vi "Fc_start_record.vi"(0 "Trace names":refnum<vi>, 1 "Start record?":refnum<vi>, 2 "Samples X Signal":u32, 3 "Global Mode":enum32{"Item 0", "Item 1"}(ring), 5 "Refresh \ntime (ms)":i32, 7 "total samples?":refnum<vi>, 9 "status+start record":bool, 11 "error in (no error)":errorcluster, 14 "Class TCP in":T1) -> (4 "Class TCP out":T1, 15 "error out":errorcluster)   [LabVIEW 2021]
doc: "This function starts the record of the signals in the application."
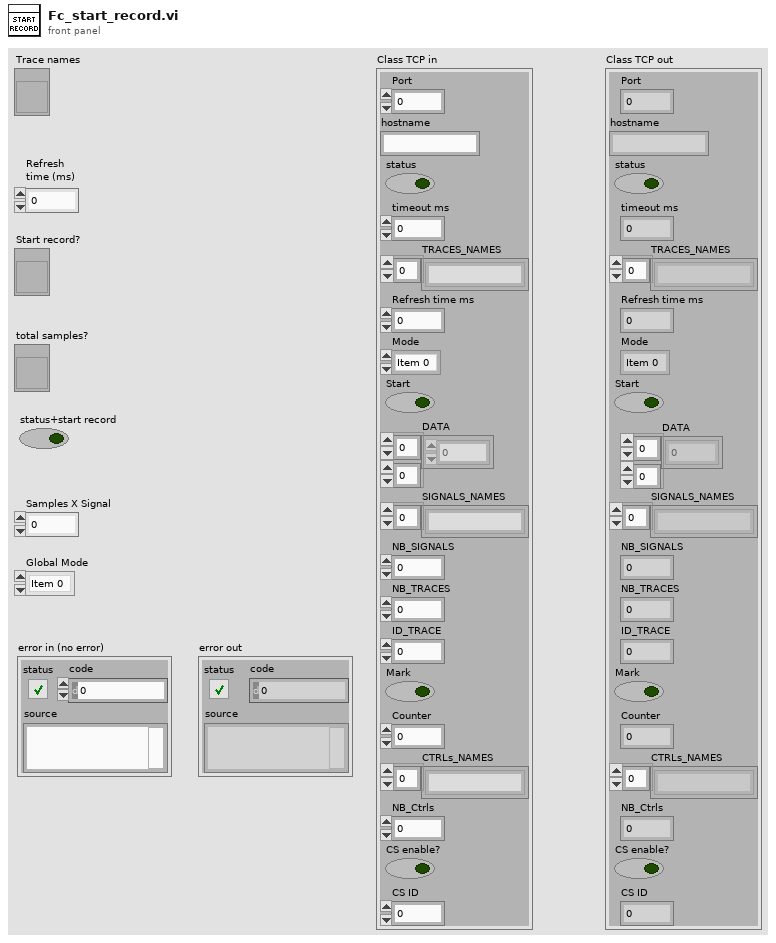
[diagram p1: front panel]
types:
  T1 = cluster{"Port":i32, "hostname":string, "status":bool, "timeout ms":i32, "TRACES_NAMES":string[], "Refresh time ms":i32, "Mode":enum32{"Item 0", "Item 1"}, "Start":bool, "DATA":sgl[][], "SIGNALS_NAMES":string[], "NB_SIGNALS":i32, "NB_TRACES":i32, "ID_TRACE":i32, "Mark":bool, "Counter":i32, "CTRLs_NAMES":string[], "NB_Ctrls":i32, "CS enable?":bool, "CS ID":i32}
  T2 = cluster{"TRACE_SIZE":i32, "CS_ID":i32, "TRACE ID":i32, "CMD":i32, "DATA(M)":i32}
  T3 = cluster{"timeout ms":i32, "remote port":u16, "Address":string}
  T4 = cluster{"SIZE":i32, " TRACE DATA":sgl[], "TRACE_SIZE":i32, "NB_TRACES":i32, "NB_TRACED_SIGNALS":i32, "NAMES TRACED SIGNALS":string[], "NAMES TRACES":string[], "CS STATUS":i32, "NB_CSs":i32, "NAMES CSs":string[], "DATA (M)":sgl[], "CMD":i32}
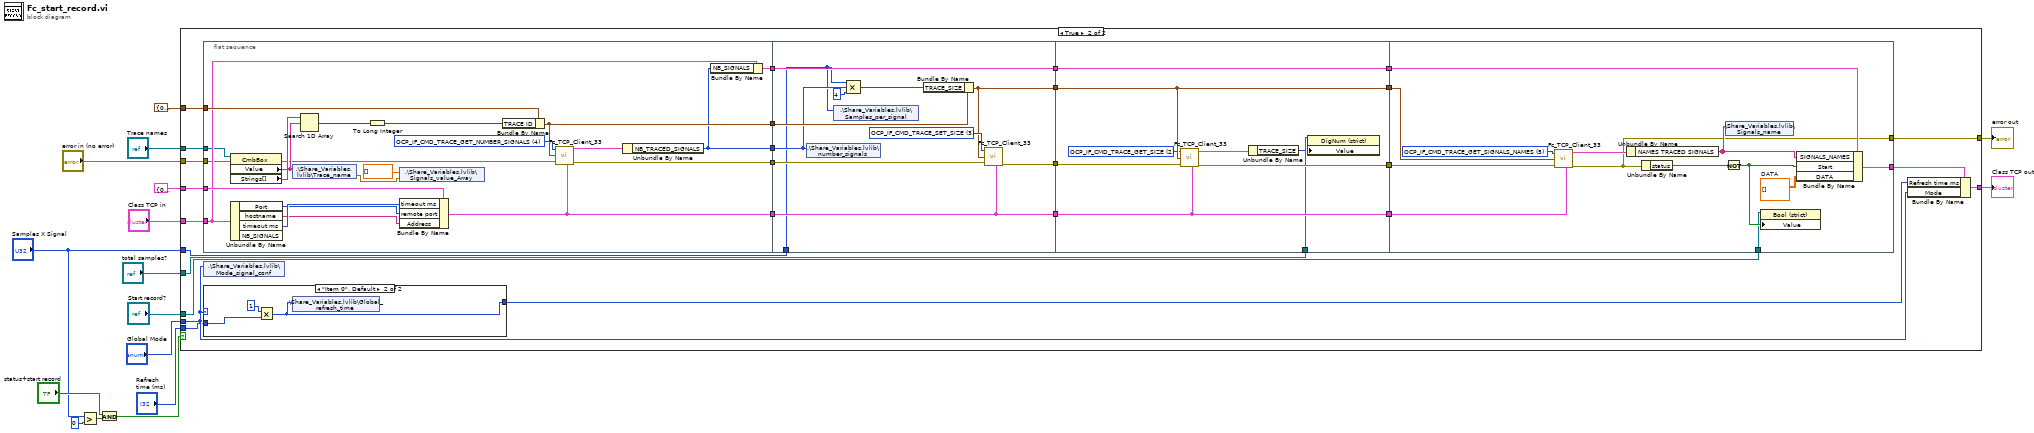
[diagram p0: block diagram]
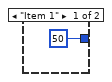
[diagram p3: hidden frame]
diagram:
  n1 = Greater?(x="Samples X Signal", y=0) -> (0:w2:bool)
  n2 = And(x="status+start record", y=w2) -> (x .and. y?=w1:bool)
  n3 = case shown="True" w1 {
    tunnel: "Class TCP in" -> [w18 w43]
    tunnel: [w18 w45] -> w12
    tunnel: T3 {"timeout ms"=0, "remote port"=0, "Address"=""} ("Comunication Cluster") -> [_ w41]
    tunnel: T2 {"TRACE_SIZE"=0, "CS_ID"=0, "TRACE ID"=0, "CMD"=0, "DATA(M)"=0} ("Input Cluster") -> [_ w40]
    tunnel: "Samples X Signal" -> [_ w39]
    tunnel: "Global Mode" -> [_ w38]
    tunnel: "Refresh \ntime (ms)" -> [_ w37]
    tunnel: "Trace names" -> [_ w36]
    tunnel: "Start record?" -> [_ w35]
    tunnel: "total samples?" -> [_ w34]
    tunnel: [w17 w33] -> w7
    tunnel: "error in (no error)" -> [w17 w32]
    frame False {
    }
    frame True {
      n4 = flat-sequence {
        tunnel: w43 -> [w51]
        tunnel: [w64] -> w31
        tunnel: [w50] -> w30
        tunnel: [w58] -> w29
        tunnel: [w53] -> w28
        tunnel: w41 -> [w57]
        tunnel: w40 -> [w56]
        tunnel: [w49] -> w27
        tunnel: w36 -> [w47]
        tunnel: w32 -> [w46]
        tunnel: w31 -> [w77]
        tunnel: [w76] -> w26
        tunnel: w30 -> [w78]
        tunnel: [w78] -> w25
        tunnel: w29 -> [w73]
        tunnel: w28 -> [w74]
        tunnel: [w74] -> w24
        tunnel: w27 -> [w72]
        tunnel: w39 -> [w68]
        tunnel: [w69] -> w23
        tunnel: w26 -> [w86]
        tunnel: [w85] -> w21
        tunnel: w25 -> [w87]
        tunnel: [w87] -> w22
        tunnel: [w84] -> w19
        tunnel: w24 -> [w83]
        tunnel: [w83] -> w20
        tunnel: w23 -> [w84]
        tunnel: w34 -> [w82]
        tunnel: w22 -> [w100]
        tunnel: [w99] -> w42
        tunnel: w21 -> [w97]
        tunnel: w20 -> [w95]
        tunnel: w19 -> [w94]
        tunnel: w35 -> [w89]
        tunnel: [w88] -> w33
        frame #0 {
          w63 = 4 items=["OCP_IF_CMD_TRACE_READ", "OCP_IF_CMD_TRACE_RESET", "OCP_IF_CMD_TRACE_GET_SIZE", "OCP_IF_CMD_TRACE_SET_SIZE", "OCP_IF_CMD_TRACE_GET_NUMBER_SIGNALS", "OCP_IF_CMD_TRACE_GET_SIGNALS_NAMES", "OCP_IF_CMD_TRACE_GET_NUMBER_TRACES", "OCP_IF_CMD_TRACE_GET_TRACES_NAMES", "OCP_IF_CMD_TRACE_GET_ADDRESS", "OCP_IF_CMD_CS_STATUS", "OCP_IF_CMD_CS_ENABLE", "OCP_IF_CMD_CS_DISABLE", "OCP_IF_CMD_CS_CONTROLLER_IF", "OCP_IF_CMD_CS_HARDWARE_IF", "OCP_IF_CMD_CS_GET_NUMBER_CONTROLLERS", "OCP_IF_CMD_CS_GET_CONTROLLERS_NAMES", "OCP_IF_CMD_PLATFORM_ID", "OCP_IF_CMD_PLATFORM_IF", "OCP_IF_CMD_OPIL_UPDATE_MEASUREMENTS", "OCP_IF_CMD_OPIL_UPDATE_SIM_DATA", "OCP_IF_CMD_OPIL_RUN_CONTROL", "OCP_IF_CMD_OPIL_INITIALIZE_CONTROL", "OCP_IF_CMD_OPIL_GET_CONTROL", "OCP_IF_CMD_OPIL_GET_CONTROLLER_DATA", "OCP_IF_CMD_END"] ("CMD")
          n5 = Unbundle By Name(w51) -> ("Port"=w61:i32, "hostname"=w60:string, "timeout ms"=w62:i32)  [unwired: 1 out]
          n6 = property on="Property Node" class="CmbBox"(reference=w47, error in=w46) -> (error out=w59:errorcluster, "Value"=w65:string, "Strings[]"=w67:string[])  [unwired: 1 out]
          n7 = shared-variable ".\\Share_Variables.lvlib\\Trace_name"(w65) -> (error out=w55:errorcluster)  [unwired: 1 in]
          n8 = Search 1D Array(1D array=w67, element=w65) -> (index of element=w66:i32)  [unwired: 1 in]
          n9 = To Long Integer(number=w66) -> (32bit integer=w48:i32)
          n10 = shared-variable ".\\Share_Variables.lvlib\\Signals_value_Array"(dbl[] [] ("Signals_value_Array"), error in=w55) -> ()  [unwired: 1 out]
          n11 = Bundle By Name(cluster=w57, "timeout ms"=w62, "remote port"=w61, "Address"=w60) -> (w53:T3)
          n12 = Bundle By Name(cluster=w56, "TRACE ID"=w48) -> (w58:T2)
          n13 = call "Fc_TCP_Client_33.vi"("CMD"=w63, "Input Cluster"=w58, "error in (no error)"=w59, "Comunication Cluster"=w53) -> ("Output cluster"=w52:T4, "error out"=w64:errorcluster)  [unwired: 4 in, 1 out]
          n14 = Unbundle By Name(w52) -> ("NB_TRACED_SIGNALS"=w49:i32)
          n15 = Bundle By Name(cluster=w51, "NB_SIGNALS"=w49) -> (w50:T1)
        }
        frame #1 {
          w75 = 3 items=["OCP_IF_CMD_TRACE_READ", "OCP_IF_CMD_TRACE_RESET", "OCP_IF_CMD_TRACE_GET_SIZE", "OCP_IF_CMD_TRACE_SET_SIZE", "OCP_IF_CMD_TRACE_GET_NUMBER_SIGNALS", "OCP_IF_CMD_TRACE_GET_SIGNALS_NAMES", "OCP_IF_CMD_TRACE_GET_NUMBER_TRACES", "OCP_IF_CMD_TRACE_GET_TRACES_NAMES", "OCP_IF_CMD_TRACE_GET_ADDRESS", "OCP_IF_CMD_CS_STATUS", "OCP_IF_CMD_CS_ENABLE", "OCP_IF_CMD_CS_DISABLE", "OCP_IF_CMD_CS_CONTROLLER_IF", "OCP_IF_CMD_CS_HARDWARE_IF", "OCP_IF_CMD_CS_GET_NUMBER_CONTROLLERS", "OCP_IF_CMD_CS_GET_CONTROLLERS_NAMES", "OCP_IF_CMD_PLATFORM_ID", "OCP_IF_CMD_PLATFORM_IF", "OCP_IF_CMD_OPIL_UPDATE_MEASUREMENTS", "OCP_IF_CMD_OPIL_UPDATE_SIM_DATA", "OCP_IF_CMD_OPIL_RUN_CONTROL", "OCP_IF_CMD_OPIL_INITIALIZE_CONTROL", "OCP_IF_CMD_OPIL_GET_CONTROL", "OCP_IF_CMD_OPIL_GET_CONTROLLER_DATA", "OCP_IF_CMD_END"] ("CMD")
          n16 = shared-variable ".\\Share_Variables.lvlib\\number_signals"(w72) -> ()  [unwired: 1 in, 1 out]
          n17 = shared-variable ".\\Share_Variables.lvlib\\Samples_per_signal"(w68) -> ()  [unwired: 1 in, 1 out]
          n18 = Compound Arithmetic op=MULTIPLY(w68, w72, 4 ("value")) -> (w70:u32)
          n19 = Bundle By Name(cluster=w73, "TRACE_SIZE"=w70) -> (w69:T2)
          n20 = call "Fc_TCP_Client_33.vi"("CMD"=w75, "Input Cluster"=w69, "error in (no error)"=w77, "Comunication Cluster"=w74) -> ("error out"=w76:errorcluster)  [unwired: 4 in, 2 out]
        }
        frame #2 {
          w80 = 2 items=["OCP_IF_CMD_TRACE_READ", "OCP_IF_CMD_TRACE_RESET", "OCP_IF_CMD_TRACE_GET_SIZE", "OCP_IF_CMD_TRACE_SET_SIZE", "OCP_IF_CMD_TRACE_GET_NUMBER_SIGNALS", "OCP_IF_CMD_TRACE_GET_SIGNALS_NAMES", "OCP_IF_CMD_TRACE_GET_NUMBER_TRACES", "OCP_IF_CMD_TRACE_GET_TRACES_NAMES", "OCP_IF_CMD_TRACE_GET_ADDRESS", "OCP_IF_CMD_CS_STATUS", "OCP_IF_CMD_CS_ENABLE", "OCP_IF_CMD_CS_DISABLE", "OCP_IF_CMD_CS_CONTROLLER_IF", "OCP_IF_CMD_CS_HARDWARE_IF", "OCP_IF_CMD_CS_GET_NUMBER_CONTROLLERS", "OCP_IF_CMD_CS_GET_CONTROLLERS_NAMES", "OCP_IF_CMD_PLATFORM_ID", "OCP_IF_CMD_PLATFORM_IF", "OCP_IF_CMD_OPIL_UPDATE_MEASUREMENTS", "OCP_IF_CMD_OPIL_UPDATE_SIM_DATA", "OCP_IF_CMD_OPIL_RUN_CONTROL", "OCP_IF_CMD_OPIL_INITIALIZE_CONTROL", "OCP_IF_CMD_OPIL_GET_CONTROL", "OCP_IF_CMD_OPIL_GET_CONTROLLER_DATA", "OCP_IF_CMD_END"] ("CMD")
          n21 = call "Fc_TCP_Client_33.vi"("CMD"=w80, "Input Cluster"=w84, "error in (no error)"=w86, "Comunication Cluster"=w83) -> ("Output cluster"=w79:T4, "error out"=w85:errorcluster)  [unwired: 4 in, 1 out]
          n22 = Unbundle By Name(w79) -> ("TRACE_SIZE"=w81:i32)
          n23 = property on="Property Node" class="DigNum (strict)"(reference=w82, "Value"=w81) -> ()  [unwired: 1 in, 2 out]
        }
        frame #3 {
          w90 = sgl[][] []  # DATA
          w96 = 5 items=["OCP_IF_CMD_TRACE_READ", "OCP_IF_CMD_TRACE_RESET", "OCP_IF_CMD_TRACE_GET_SIZE", "OCP_IF_CMD_TRACE_SET_SIZE", "OCP_IF_CMD_TRACE_GET_NUMBER_SIGNALS", "OCP_IF_CMD_TRACE_GET_SIGNALS_NAMES", "OCP_IF_CMD_TRACE_GET_NUMBER_TRACES", "OCP_IF_CMD_TRACE_GET_TRACES_NAMES", "OCP_IF_CMD_TRACE_GET_ADDRESS", "OCP_IF_CMD_CS_STATUS", "OCP_IF_CMD_CS_ENABLE", "OCP_IF_CMD_CS_DISABLE", "OCP_IF_CMD_CS_CONTROLLER_IF", "OCP_IF_CMD_CS_HARDWARE_IF", "OCP_IF_CMD_CS_GET_NUMBER_CONTROLLERS", "OCP_IF_CMD_CS_GET_CONTROLLERS_NAMES", "OCP_IF_CMD_PLATFORM_ID", "OCP_IF_CMD_PLATFORM_IF", "OCP_IF_CMD_OPIL_UPDATE_MEASUREMENTS", "OCP_IF_CMD_OPIL_UPDATE_SIM_DATA", "OCP_IF_CMD_OPIL_RUN_CONTROL", "OCP_IF_CMD_OPIL_INITIALIZE_CONTROL", "OCP_IF_CMD_OPIL_GET_CONTROL", "OCP_IF_CMD_OPIL_GET_CONTROLLER_DATA", "OCP_IF_CMD_END"] ("CMD")
          n24 = call "Fc_TCP_Client_33.vi"("CMD"=w96, "Input Cluster"=w94, "error in (no error)"=w97, "Comunication Cluster"=w95) -> ("Output cluster"=w98:T4, "error out"=w88:errorcluster)  [unwired: 4 in, 1 out]
          n25 = Unbundle By Name(w98) -> ("NAMES TRACED SIGNALS"=w92:string[])
          n26 = Unbundle By Name(w88) -> ("status"=w93:bool)
          n27 = Not(x=w93) -> (.not. x?=w91:bool)
          n28 = shared-variable ".\\Share_Variables.lvlib\\Signals_name"(w92) -> ()  [unwired: 1 in, 1 out]
          n29 = property class="Bool (strict)"(reference=w89, "Value"=w91) -> ()  [unwired: 1 in, 2 out]
          n30 = Bundle By Name(cluster=w100, "SIGNALS_NAMES"=w92, "Start"=w91, "DATA"=w90) -> (w99:T1)
        }
      }
      n31 = shared-variable ".\\Share_Variables.lvlib\\Mode_signal_conf"(w38) -> ()  [unwired: 1 in, 1 out]
      n32 = case shown="\"Item 0\", Default" w38 {
        tunnel: [50 ("Refresh time (sec)") w103] -> w44
        tunnel: w37 -> [_ w102]
        frame "Item 1" {
        }
        frame "Item 0", Default {
          n33 = Multiply(x=1, y=w102) -> (x*y=w103:i32)
          n34 = shared-variable ".\\Share_Variables.lvlib\\Global_refresh_time"(w103) -> ()  [unwired: 1 in, 1 out]
        }
      }
      n35 = Bundle By Name(cluster=w42, "Refresh time ms"=w44, "Mode"=w38) -> (w45:T1)
    }
  }
  "Class TCP out" <- w12
  "error out" <- w7
